vi "BCU参数读取-Auto.vi"(8 "CAN端口":u16(ring), 9 "设备索引号":u16(ring), 10 "CAN卡类型":u32(ring)=21, 11 "Myindex":dbl=1.0) -> (3 "成功":bool)   [LabVIEW 2013] (continued)
                      n2808 = property class="Tbl (严格)"(reference=w4454, "Active Cell"=w4453, "Cell BG Color"=u32 6618880) -> ()  [unwired: 1 in, 2 out]
                    }
                  }
                }
                n2809 = Select(t=0, s=w4406, f=1) -> (s? t:f=w4405:i32)
                n2810 = property on="从板个数" class="DigNum (严格)"("NumText.BGColor"=u32 13816530) -> ()  [unwired: 2 in, 2 out]
                n2811 = property on="项目信息" class="Tbl (严格)"("Disabled"=w4405) -> ()  [unwired: 2 in, 2 out]
                n2812 = global read "功能码全局.vi" "主板项目信息5"() -> (w4413:bool[])
                n2813 = global read "功能码全局.vi" "主板项目信息6"() -> (w4411:bool[])
                n2814 = Index Array(array=w4413, index=5 ("索引")) -> (element=w4410:bool)
                n2815 = Index Array(array=w4411, index=6 ("索引")) -> (element=w4409:bool)
                n2816 = Not(x=w4419) -> (.not. x?=w4418:bool)
              }
              frame "保险位置" {
                w4467 = 2
                w4469 = FALSE
                n2817 = property on="电池实际容量(A)" class="DigNum (严格)"("Disabled"=w4467) -> ()  [unwired: 2 in, 2 out]
                n2818 = property on="使用者" class="DigNum (严格)"("Disabled"=w4467) -> ()  [unwired: 2 in, 2 out]
                n2819 = property on="SOH(%)" class="DigNum (严格)"("Disabled"=w4467) -> ()  [unwired: 2 in, 2 out]
                n2820 = property on="电池额定容量(A)" class="DigNum (严格)"("Disabled"=w4467) -> ()  [unwired: 2 in, 2 out]
                n2821 = property on="SOC(%)" class="DigNum (严格)"("Disabled"=w4467) -> ()  [unwired: 2 in, 2 out]
                n2822 = local read "从板个数"() -> (w4465:dbl)
                n2823 = property on="系统时钟" class="Str"("Disabled"=w4467) -> ()  [unwired: 2 in, 2 out]
                n2824 = property on="配置文件版本" class="Str"("Disabled"=w4467) -> ()  [unwired: 2 in, 2 out]
                n2825 = property on="车架(牌)号" class="Str"("Disabled"=w4467) -> ()  [unwired: 2 in, 2 out]
                n2826 = property on="产品编号" class="Str"("Disabled"=w4467) -> ()  [unwired: 2 in, 2 out]
                n2827 = control-ref of="项目信息"() -> (w4466:refnum<vi>)
                n2828 = stacked-sequence {
                  tunnel: w4466 -> [w4478 w4481]
                  tunnel: w4465 -> [w4471 w4480]
                  frame #0 {
                    n2829 = Multiply(x=w4471, y=4.0) -> (x*y=w4473:dbl)
                    n2830 = Compound Arithmetic op=ADD(24.0 ("值"), w4473) -> (w4475:dbl)
                    n2831 = Bundle(w4475, 0) -> (w4477:cluster{dbl, i32})  [unwired: 1 out]
                    n2832 = property class="Tbl (严格)"(reference=w4478, "Index Values"=w4477) -> ()  [unwired: 1 in, 2 out]
                  }
                  frame #1 {
                    n2833 = for {
                      N: 20 -> [_]
                      tunnel: w4481 -> [w4491]
                      tunnel: w4480 -> [w4486]
                      i -> [w4485]
                      n2834 = Multiply(x=4.0, y=w4486) -> (x*y=w4483:dbl)
                      n2835 = Compound Arithmetic op=ADD(24.0 ("值"), w4483, w4485) -> (w4488:dbl)
                      n2836 = Bundle(w4488, 0) -> (w4490:cluster{dbl, i32})  [unwired: 1 out]
                      n2837 = property class="Tbl (严格)"(reference=w4491, "Active Cell"=w4490, "Cell BG Color"=u32 6618880) -> ()  [unwired: 1 in, 2 out]
                    }
                  }
                }
                n2838 = property on="从板个数" class="DigNum (严格)"("NumText.BGColor"=u32 13816530) -> ()  [unwired: 2 in, 2 out]
                n2839 = Select(t=0, s=w4458, f=1) -> (s? t:f=w4456:i32)
                n2840 = global read "功能码全局.vi" "主板项目信息4"() -> (w4463:bool[])
                n2841 = property on="项目信息" class="Tbl (严格)"("Disabled"=w4456) -> ()  [unwired: 2 in, 2 out]
                n2842 = Index Array(array=w4463, index #1=5 ("索引"), index #2=6 ("索引")) -> (element #1=w4461:bool, element #2=w4460:bool)
                n2843 = Not(x=w4469) -> (.not. x?=w4468:bool)
              }
              frame "SOC" {
                w4502 = 2
                w4504 = FALSE
                n2844 = property on="电池实际容量(A)" class="DigNum (严格)"("Disabled"=w4502) -> ()  [unwired: 2 in, 2 out]
                n2845 = property on="使用者" class="DigNum (严格)"("Disabled"=w4502) -> ()  [unwired: 2 in, 2 out]
                n2846 = property on="SOH(%)" class="DigNum (严格)"("Disabled"=w4502) -> ()  [unwired: 2 in, 2 out]
                n2847 = property on="电池额定容量(A)" class="DigNum (严格)"("Disabled"=w4502) -> ()  [unwired: 2 in, 2 out]
                n2848 = property on="从板个数" class="DigNum (严格)"("NumText.BGColor"=u32 13816530) -> ()  [unwired: 2 in, 2 out]
                n2849 = property on="系统时钟" class="Str"("Disabled"=w4502) -> ()  [unwired: 2 in, 2 out]
                n2850 = property on="配置文件版本" class="Str"("Disabled"=w4502) -> ()  [unwired: 2 in, 2 out]
                n2851 = property on="车架(牌)号" class="Str"("Disabled"=w4502) -> ()  [unwired: 2 in, 2 out]
                n2852 = property on="项目信息" class="Tbl (严格)"("Disabled"=w4502) -> ()  [unwired: 2 in, 2 out]
                n2853 = property on="产品编号" class="Str"("Disabled"=w4502) -> ()  [unwired: 2 in, 2 out]
                n2854 = Select(t=0, s=w4494, f=0) -> (s? t:f=w4493:i32)
                n2855 = property on="SOC(%)" class="DigNum (严格)"("Disabled"=w4493) -> ()  [unwired: 2 in, 2 out]
                n2856 = property on="项目信息2" class="Clust (严格)"("DisabledEnum"=w4493) -> ()  [unwired: 2 in, 2 out]
                n2857 = global read "功能码全局.vi" "主板项目信息7"() -> (w4500:bool[])
                n2858 = Index Array(array=w4500, index #1=2 ("索引"), index #2=5 ("索引")) -> (element #1=w4498:bool, element #2=w4497:bool)
                n2859 = Not(x=w4504) -> (.not. x?=w4503:bool)
              }
              frame "电池额定实际容量" {
                w4516 = 2
                w4518 = FALSE
                n2860 = property on="使用者" class="DigNum (严格)"("Disabled"=w4516) -> ()  [unwired: 2 in, 2 out]
                n2861 = property on="SOH(%)" class="DigNum (严格)"("Disabled"=w4516) -> ()  [unwired: 2 in, 2 out]
                n2862 = property on="SOC(%)" class="DigNum (严格)"("Disabled"=w4516) -> ()  [unwired: 2 in, 2 out]
                n2863 = property on="从板个数" class="DigNum (严格)"("NumText.BGColor"=u32 13816530) -> ()  [unwired: 2 in, 2 out]
                n2864 = property on="系统时钟" class="Str"("Disabled"=w4516) -> ()  [unwired: 2 in, 2 out]
                n2865 = property on="配置文件版本" class="Str"("Disabled"=w4516) -> ()  [unwired: 2 in, 2 out]
                n2866 = property on="车架(牌)号" class="Str"("Disabled"=w4516) -> ()  [unwired: 2 in, 2 out]
                n2867 = property on="项目信息" class="Tbl (严格)"("Disabled"=w4516) -> ()  [unwired: 2 in, 2 out]
                n2868 = property on="产品编号" class="Str"("Disabled"=w4516) -> ()  [unwired: 2 in, 2 out]
                n2869 = Select(t=0, s=w4508, f=1) -> (s? t:f=w4507:i32)
                n2870 = property on="电池实际容量(A)" class="DigNum (严格)"("Disabled"=w4507) -> ()  [unwired: 2 in, 2 out]
                n2871 = property on="电池额定容量(A)" class="DigNum (严格)"("Disabled"=w4507) -> ()  [unwired: 2 in, 2 out]
                n2872 = property on="项目信息2" class="Clust (严格)"("DisabledEnum"=w4507) -> ()  [unwired: 2 in, 2 out]
                n2873 = global read "功能码全局.vi" "主板项目信息7"() -> (w4514:bool[])
                n2874 = Index Array(array=w4514, index #1=3 ("索引"), index #2=6 ("索引")) -> (element #1=w4512:bool, element #2=w4511:bool)
                n2875 = Not(x=w4518) -> (.not. x?=w4517:bool)
              }
              frame "配置文件版本" {
                w4531 = 2
                w4533 = FALSE
                n2876 = property on="使用者" class="DigNum (严格)"("Disabled"=w4531) -> ()  [unwired: 2 in, 2 out]
                n2877 = property on="SOH(%)" class="DigNum (严格)"("Disabled"=w4531) -> ()  [unwired: 2 in, 2 out]
                n2878 = property on="SOC(%)" class="DigNum (严格)"("Disabled"=w4531) -> ()  [unwired: 2 in, 2 out]
                n2879 = property on="电池实际容量(A)" class="DigNum (严格)"("Disabled"=w4531) -> ()  [unwired: 2 in, 2 out]
                n2880 = property on="从板个数" class="DigNum (严格)"("NumText.BGColor"=u32 13816530) -> ()  [unwired: 2 in, 2 out]
                n2881 = property on="电池额定容量(A)" class="DigNum (严格)"("Disabled"=w4531) -> ()  [unwired: 2 in, 2 out]
                n2882 = property on="系统时钟" class="Str"("Disabled"=w4531) -> ()  [unwired: 2 in, 2 out]
                n2883 = property on="车架(牌)号" class="Str"("Disabled"=w4531) -> ()  [unwired: 2 in, 2 out]
                n2884 = property on="项目信息" class="Tbl (严格)"("Disabled"=w4531) -> ()  [unwired: 2 in, 2 out]
                n2885 = property on="产品编号" class="Str"("Disabled"=w4531) -> ()  [unwired: 2 in, 2 out]
                n2886 = Select(t=0, s=w4522, f=1) -> (s? t:f=w4521:i32)
                n2887 = property on="项目信息2" class="Clust (严格)"("DisabledEnum"=w4521) -> ()  [unwired: 2 in, 2 out]
                n2888 = property on="配置文件版本" class="Str"("Disabled"=w4521) -> ()  [unwired: 2 in, 2 out]
                n2889 = global read "功能码全局.vi" "主板项目信息5"() -> (w4529:bool[])
                n2890 = global read "功能码全局.vi" "主板项目信息6"() -> (w4528:bool[])
                n2891 = Index Array(array=w4529, index=6 ("索引")) -> (element=w4526:bool)
                n2892 = Index Array(array=w4528, index=7 ("索引")) -> (element=w4525:bool)
                n2893 = Not(x=w4533) -> (.not. x?=w4532:bool)
              }
              frame "参数修改记录" {
                w4546 = 2
                w4548 = FALSE
                n2894 = property on="SOH(%)" class="DigNum (严格)"("Disabled"=w4546) -> ()  [unwired: 2 in, 2 out]
                n2895 = property on="SOC(%)" class="DigNum (严格)"("Disabled"=w4546) -> ()  [unwired: 2 in, 2 out]
                n2896 = property on="电池实际容量(A)" class="DigNum (严格)"("Disabled"=w4546) -> ()  [unwired: 2 in, 2 out]
                n2897 = property on="电池额定容量(A)" class="DigNum (严格)"("Disabled"=w4546) -> ()  [unwired: 2 in, 2 out]
                n2898 = property on="从板个数" class="DigNum (严格)"("NumText.BGColor"=u32 13816530) -> ()  [unwired: 2 in, 2 out]
                n2899 = property on="系统时钟" class="Str"("Disabled"=w4546) -> ()  [unwired: 2 in, 2 out]
                n2900 = property on="车架(牌)号" class="Str"("Disabled"=w4546) -> ()  [unwired: 2 in, 2 out]
                n2901 = property on="配置文件版本" class="Str"("Disabled"=w4546) -> ()  [unwired: 2 in, 2 out]
                n2902 = property on="项目信息" class="Tbl (严格)"("Disabled"=w4546) -> ()  [unwired: 2 in, 2 out]
                n2903 = property on="产品编号" class="Str"("Disabled"=w4546) -> ()  [unwired: 2 in, 2 out]
                n2904 = Select(t=0, s=w4537, f=1) -> (s? t:f=w4536:i32)
                n2905 = property on="使用者" class="DigNum (严格)"("Disabled"=w4536) -> ()  [unwired: 2 in, 2 out]
                n2906 = property on="项目信息2" class="Clust (严格)"("DisabledEnum"=w4536) -> ()  [unwired: 2 in, 2 out]
                n2907 = global read "功能码全局.vi" "主板项目信息7"() -> (w4543:bool[])
                n2908 = global read "功能码全局.vi" "主板项目信息5"() -> (w4544:bool[])
                n2909 = Index Array(array=w4543, index=0 ("索引")) -> (element=w4541:bool)
                n2910 = Index Array(array=w4544, index=7 ("索引")) -> (element=w4540:bool)
                n2911 = Not(x=w4548) -> (.not. x?=w4547:bool)
              }
              frame "车牌号" {
                w4561 = 2
                w4563 = FALSE
                n2912 = property on="SOH(%)" class="DigNum (严格)"("Disabled"=w4561) -> ()  [unwired: 2 in, 2 out]
                n2913 = property on="使用者" class="DigNum (严格)"("Disabled"=w4561) -> ()  [unwired: 2 in, 2 out]
                n2914 = property on="SOC(%)" class="DigNum (严格)"("Disabled"=w4561) -> ()  [unwired: 2 in, 2 out]
                n2915 = property on="电池实际容量(A)" class="DigNum (严格)"("Disabled"=w4561) -> ()  [unwired: 2 in, 2 out]
                n2916 = property on="电池额定容量(A)" class="DigNum (严格)"("Disabled"=w4561) -> ()  [unwired: 2 in, 2 out]
                n2917 = property on="从板个数" class="DigNum (严格)"("NumText.BGColor"=u32 13816530) -> ()  [unwired: 2 in, 2 out]
                n2918 = property on="系统时钟" class="Str"("Disabled"=w4561) -> ()  [unwired: 2 in, 2 out]
                n2919 = property on="配置文件版本" class="Str"("Disabled"=w4561) -> ()  [unwired: 2 in, 2 out]
                n2920 = property on="项目信息" class="Tbl (严格)"("Disabled"=w4561) -> ()  [unwired: 2 in, 2 out]
                n2921 = property on="产品编号" class="Str"("Disabled"=w4561) -> ()  [unwired: 2 in, 2 out]
                n2922 = Select(t=0, s=w4552, f=1) -> (s? t:f=w4551:i32)
                n2923 = property on="车架(牌)号" class="Str"("Disabled"=w4551) -> ()  [unwired: 2 in, 2 out]
                n2924 = property on="项目信息2" class="Clust (严格)"("DisabledEnum"=w4551) -> ()  [unwired: 2 in, 2 out]
                n2925 = global read "功能码全局.vi" "主板项目信息7"() -> (w4558:bool[])
                n2926 = global read "功能码全局.vi" "主板项目信息6"() -> (w4559:bool[])
                n2927 = Index Array(array=w4558, index=1 ("索引")) -> (element=w4556:bool)
                n2928 = Index Array(array=w4559, index=0 ("索引")) -> (element=w4555:bool)
                n2929 = Not(x=w4563) -> (.not. x?=w4562:bool)
              }
              frame "SOH" {
                w4575 = 2
                w4577 = FALSE
                n2930 = property on="使用者" class="DigNum (严格)"("Disabled"=w4575) -> ()  [unwired: 2 in, 2 out]
                n2931 = property on="SOC(%)" class="DigNum (严格)"("Disabled"=w4575) -> ()  [unwired: 2 in, 2 out]
                n2932 = property on="电池实际容量(A)" class="DigNum (严格)"("Disabled"=w4575) -> ()  [unwired: 2 in, 2 out]
                n2933 = property on="电池额定容量(A)" class="DigNum (严格)"("Disabled"=w4575) -> ()  [unwired: 2 in, 2 out]
                n2934 = property on="从板个数" class="DigNum (严格)"("NumText.BGColor"=u32 13816530) -> ()  [unwired: 2 in, 2 out]
                n2935 = property on="系统时钟" class="Str"("Disabled"=w4575) -> ()  [unwired: 2 in, 2 out]
                n2936 = property on="配置文件版本" class="Str"("Disabled"=w4575) -> ()  [unwired: 2 in, 2 out]
                n2937 = property on="项目信息" class="Tbl (严格)"("Disabled"=w4575) -> ()  [unwired: 2 in, 2 out]
                n2938 = property on="产品编号" class="Str"("Disabled"=w4575) -> ()  [unwired: 2 in, 2 out]
                n2939 = property on="车架(牌)号" class="Str"("Disabled"=w4575) -> ()  [unwired: 2 in, 2 out]
                n2940 = Select(t=0, s=w4567, f=1) -> (s? t:f=w4566:i32)
                n2941 = property on="项目信息2" class="Clust (严格)"("DisabledEnum"=w4566) -> ()  [unwired: 2 in, 2 out]
                n2942 = property on="SOH(%)" class="DigNum (严格)"("Disabled"=w4566) -> ()  [unwired: 2 in, 2 out]
                n2943 = global read "功能码全局.vi" "主板项目信息7"() -> (w4574:bool[])
                n2944 = Index Array(array=w4574, index #1=4 ("索引"), index #2=7 ("索引")) -> (element #1=w4571:bool, element #2=w4570:bool)
                n2945 = Not(x=w4577) -> (.not. x?=w4576:bool)
              }
              frame "SOC过低(2)", "SOC过高(2)", "SOH过低(2)", "充电电流过高(2)", "单体电压过低(2)", "单体电压过高(2)", "单组电压不均衡(2)", "单组温度不均衡(2)", "二级故障阀值", "放电电流过高(2)", "极柱温度过高(2)", "内阻过大(2)", "温度过低(2)", "温度过高(2)", "整组电压不均衡(2)", "整组温度不均衡(2)", "总电压过低(2)", "总电压过高(2)" {
                w4589 = FALSE
                n2946 = property on="从板个数" class="DigNum (严格)"("NumText.BGColor"=u32 13816530) -> ()  [unwired: 2 in, 2 out]
                n2947 = Select(t=0, s=w4581, f=1) -> (s? t:f=w4580:i32)
                n2948 = property on="一级故障 2" class="Clust (严格)"("DisabledEnum"=w4580) -> ()  [unwired: 2 in, 2 out]
                n2949 = global read "功能码全局.vi" "主板故障阀值9"() -> (w4587:bool[])
                n2950 = Index Array(array=w4587, index #1=3 ("索引"), index #2=6 ("索引")) -> (element #1=w4585:bool, element #2=w4584:bool)
                n2951 = Not(x=w4589) -> (.not. x?=w4590:bool)
              }
              frame "SOC过低(3)", "SOC过高(3)", "SOH过低(3)", "充电电流过高(3)", "单体电压过低(3)", "单体电压过高(3)", "单组电压不均衡(3)", "单组温度不均衡(3)", "放电电流过高(3)", "极柱温度过高(3)", "内阻过大(3)", "三级故障阀值", "温度过低(3)", "温度过高(3)", "整组电压不均衡(3)", "整组温度不均衡(3)", "总电压过低(3)", "总电压过高(3)" {
                w4603 = FALSE
                n2952 = property on="从板个数" class="DigNum (严格)"("NumText.BGColor"=u32 13816530) -> ()  [unwired: 2 in, 2 out]
                n2953 = Select(t=0, s=w4594, f=1) -> (s? t:f=w4593:i32)
                n2954 = property on="一级故障 3" class="Clust (严格)"("DisabledEnum"=w4593) -> ()  [unwired: 2 in, 2 out]
                n2955 = global read "功能码全局.vi" "主板故障阀值9"() -> (w4600:bool[])
                n2956 = Index Array(array=w4600, index #1=4 ("索引"), index #2=7 ("索引")) -> (element #1=w4598:bool, element #2=w4597:bool)
                n2957 = Not(x=w4603) -> (.not. x?=w4602:bool)
              }
              frame "SOC过低", "SOC过高", "SOH过低", "充电电流过高", "单体电压过低", "单体电压过高", "单组电压不均衡", "单组温度不均衡", "放电电流过高", "极柱温度过高", "内阻过大", "温度过低", "温度过高", "一级故障阀值", "整组电压不均衡", "整组温度不均衡", "总电压过低", "总电压过高" {
                w4616 = FALSE
                n2958 = Select(t=0, s=w4607, f=1) -> (s? t:f=w4606:i32)
                n2959 = property on="从板个数" class="DigNum (严格)"("NumText.BGColor"=u32 13816530) -> ()  [unwired: 2 in, 2 out]
                n2960 = property on="一级故障" class="Clust (严格)"("DisabledEnum"=w4606) -> ()  [unwired: 2 in, 2 out]
                n2961 = global read "功能码全局.vi" "主板故障阀值9"() -> (w4613:bool[])
                n2962 = Index Array(array=w4613, index #1=2 ("索引"), index #2=5 ("索引")) -> (element #1=w4611:bool, element #2=w4610:bool)
                n2963 = Not(x=w4616) -> (.not. x?=w4615:bool)
              }
              frame "充电控制参数", "电流步长", "最大允许充电电流", "最大允许充电温度", "最大允许单体电压", "最大允许总电压", "最小允许充电电流", "最小允许充电温度", "最小允许单体电压" {
                w4619 = 2
                w4630 = FALSE
                n2964 = property on="从板个数" class="DigNum (严格)"("NumText.BGColor"=u32 13816530) -> ()  [unwired: 2 in, 2 out]
                n2965 = property on="风机开启温度" class="DigNum (严格)"("Disabled"=w4619) -> ()  [unwired: 2 in, 2 out]
                n2966 = property on="风机关闭温度" class="DigNum (严格)"("Disabled"=w4619) -> ()  [unwired: 2 in, 2 out]
                n2967 = property on="加热开启温度" class="DigNum (严格)"("Disabled"=w4619) -> ()  [unwired: 2 in, 2 out]
                n2968 = property on="加热关闭温度" class="DigNum (严格)"("Disabled"=w4619) -> ()  [unwired: 2 in, 2 out]
                n2969 = property on="风机开启温差" class="DigNum (严格)"("Disabled"=w4619) -> ()  [unwired: 2 in, 2 out]
                n2970 = property on="风机关闭温差" class="DigNum (严格)"("Disabled"=w4619) -> ()  [unwired: 2 in, 2 out]
                n2971 = property on="加热控制参数" class="Clust (严格)"("DisabledEnum"=w4619) -> ()  [unwired: 2 in, 2 out]
                n2972 = Select(t=0, s=w4621, f=1) -> (s? t:f=w4620:i32)
                n2973 = property on="最大允许总电压" class="DigNum (严格)"("Disabled"=w4620) -> ()  [unwired: 2 in, 2 out]
                n2974 = property on="最大允许充电温度" class="DigNum (严格)"("Disabled"=w4620) -> ()  [unwired: 2 in, 2 out]
                n2975 = property on="最小允许充电温度" class="DigNum (严格)"("Disabled"=w4620) -> ()  [unwired: 2 in, 2 out]
                n2976 = property on="电流步长" class="DigNum (严格)"("Disabled"=w4620) -> ()  [unwired: 2 in, 2 out]
                n2977 = property on="最大允许单体电压" class="DigNum (严格)"("Disabled"=w4620) -> ()  [unwired: 2 in, 2 out]
                n2978 = property on="最小允许单体电压" class="DigNum (严格)"("Disabled"=w4620) -> ()  [unwired: 2 in, 2 out]
                n2979 = property on="最大允许充电电流" class="DigNum (严格)"("Disabled"=w4620) -> ()  [unwired: 2 in, 2 out]
                n2980 = property on="最小允许充电电流" class="DigNum (严格)"("Disabled"=w4620) -> ()  [unwired: 2 in, 2 out]
                n2981 = global read "功能码全局.vi" "主板控制类信息10"() -> (w4627:bool[])
                n2982 = Index Array(array=w4627, index #1=5 ("索引"), index #2=7 ("索引")) -> (element #1=w4625:bool, element #2=w4624:bool)
                n2983 = Not(x=w4630) -> (.not. x?=w4629:bool)
              }
              frame "风机关闭温差", "风机关闭温度", "风机开启温差", "风机开启温度", "加热关闭温差", "加热关闭温度", "加热开启温度", "加热控制参数" {
                w4642 = 2
                w4644 = FALSE
                n2984 = Select(t=0, s=w4634, f=1) -> (s? t:f=w4633:i32)
                n2985 = property on="从板个数" class="DigNum (严格)"("NumText.BGColor"=u32 13816530) -> ()  [unwired: 2 in, 2 out]
                n2986 = property on="加热控制参数" class="Clust (严格)"("DisabledEnum"=w4633) -> ()  [unwired: 2 in, 2 out]
                n2987 = property on="风机开启温度" class="DigNum (严格)"("Disabled"=w4633) -> ()  [unwired: 2 in, 2 out]
                n2988 = property on="风机关闭温度" class="DigNum (严格)"("Disabled"=w4633) -> ()  [unwired: 2 in, 2 out]
                n2989 = property on="加热开启温度" class="DigNum (严格)"("Disabled"=w4633) -> ()  [unwired: 2 in, 2 out]
                n2990 = property on="加热关闭温度" class="DigNum (严格)"("Disabled"=w4633) -> ()  [unwired: 2 in, 2 out]
                n2991 = property on="风机开启温差" class="DigNum (严格)"("Disabled"=w4633) -> ()  [unwired: 2 in, 2 out]
                n2992 = property on="风机关闭温差" class="DigNum (严格)"("Disabled"=w4633) -> ()  [unwired: 2 in, 2 out]
                n2993 = property on="最大允许总电压" class="DigNum (严格)"("Disabled"=w4642) -> ()  [unwired: 2 in, 2 out]
                n2994 = property on="最大允许充电温度" class="DigNum (严格)"("Disabled"=w4642) -> ()  [unwired: 2 in, 2 out]
                n2995 = property on="最小允许充电温度" class="DigNum (严格)"("Disabled"=w4642) -> ()  [unwired: 2 in, 2 out]
                n2996 = property on="电流步长" class="DigNum (严格)"("Disabled"=w4642) -> ()  [unwired: 2 in, 2 out]
                n2997 = property on="最大允许单体电压" class="DigNum (严格)"("Disabled"=w4642) -> ()  [unwired: 2 in, 2 out]
                n2998 = property on="最小允许单体电压" class="DigNum (严格)"("Disabled"=w4642) -> ()  [unwired: 2 in, 2 out]
                n2999 = property on="最大允许充电电流" class="DigNum (严格)"("Disabled"=w4642) -> ()  [unwired: 2 in, 2 out]
                n3000 = property on="最小允许充电电流" class="DigNum (严格)"("Disabled"=w4642) -> ()  [unwired: 2 in, 2 out]
                n3001 = global read "功能码全局.vi" "主板控制类信息10"() -> (w4640:bool[])
                n3002 = Index Array(array=w4640, index #1=4 ("索引"), index #2=6 ("索引")) -> (element #1=w4638:bool, element #2=w4637:bool)
                n3003 = Not(x=w4644) -> (.not. x?=w4643:bool)
              }
              frame "电池信息" {
                w4657 = FALSE
                n3004 = Select(t=0, s=w4648, f=1) -> (s? t:f=w4647:i32)
                n3005 = property on="电池串联" class="DigNum (严格)"("Disabled"=w4647) -> ()  [unwired: 2 in, 2 out]
                n3006 = property on="电池并联" class="DigNum (严格)"("Disabled"=w4647) -> ()  [unwired: 2 in, 2 out]
                n3007 = property on="电池包额定容量" class="DigNum (严格)"("Disabled"=w4647) -> ()  [unwired: 2 in, 2 out]
                n3008 = property on="电池包额定能量(kWh)" class="DigNum (严格)"("Disabled"=w4647) -> ()  [unwired: 2 in, 2 out]
                n3009 = property on="电池包额定总电压" class="DigNum (严格)"("Disabled"=w4647) -> ()  [unwired: 2 in, 2 out]
                n3010 = property on="实际容量" class="DigNum (严格)"("Disabled"=w4647) -> ()  [unwired: 2 in, 2 out]
                n3011 = property on="电池包组号" class="Str"("Disabled"=w4647) -> ()  [unwired: 2 in, 2 out]
                n3012 = property on="电池生产日期" class="Str"("Disabled"=w4647) -> ()  [unwired: 2 in, 2 out]
                n3013 = property on="电池厂家" class="Str"("Disabled"=w4647) -> ()  [unwired: 2 in, 2 out]
                n3014 = property on="电池类型" class="Str"("Disabled"=w4647) -> ()  [unwired: 2 in, 2 out]
                n3015 = property on="累计充电总安时" class="DigNum (严格)"("Disabled"=w4647) -> ()  [unwired: 2 in, 2 out]
                n3016 = property on="累计放电总安时" class="DigNum (严格)"("Disabled"=w4647) -> ()  [unwired: 2 in, 2 out]
                n3017 = property on="电池放空次数" class="DigNum (严格)"("Disabled"=w4647) -> ()  [unwired: 2 in, 2 out]
                n3018 = property on="电池充满次数" class="DigNum (严格)"("Disabled"=w4647) -> ()  [unwired: 2 in, 2 out]
                n3019 = property on="电池充电次数" class="DigNum (严格)"("Disabled"=w4647) -> ()  [unwired: 2 in, 2 out]
                n3020 = property on="电池信息" class="Clust (严格)"("DisabledEnum"=w4647) -> ()  [unwired: 2 in, 2 out]
                n3021 = global read "功能码全局.vi" "主板版本号11"() -> (w4654:bool[])
                n3022 = property on="从板个数" class="DigNum (严格)"("NumText.BGColor"=u32 13816530) -> ()  [unwired: 2 in, 2 out]
                n3023 = Index Array(array=w4654, index #1=0 ("索引"), index #2=1 ("索引")) -> (element #1=w4652:bool, element #2=w4651:bool)
                n3024 = Not(x=w4657) -> (.not. x?=w4656:bool)
              }
              frame "电池信息1" {
                w4669 = 2
                w4671 = FALSE
                n3025 = Select(t=0, s=w4661, f=1) -> (s? t:f=w4660:i32)
                n3026 = property on="电池信息" class="Clust (严格)"("DisabledEnum"=w4660) -> ()  [unwired: 2 in, 2 out]
                n3027 = property on="电池生产日期" class="Str"("Disabled"=w4660) -> ()  [unwired: 2 in, 2 out]
                n3028 = property on="电池厂家" class="Str"("Disabled"=w4660) -> ()  [unwired: 2 in, 2 out]
                n3029 = property on="电池类型" class="Str"("Disabled"=w4660) -> ()  [unwired: 2 in, 2 out]
                n3030 = property on="电池串联" class="DigNum (严格)"("Disabled"=w4660) -> ()  [unwired: 2 in, 2 out]
                n3031 = property on="电池并联" class="DigNum (严格)"("Disabled"=w4660) -> ()  [unwired: 2 in, 2 out]
                n3032 = property on="电池包额定容量" class="DigNum (严格)"("Disabled"=w4660) -> ()  [unwired: 2 in, 2 out]
                n3033 = property on="电池包额定能量(kWh)" class="DigNum (严格)"("Disabled"=w4660) -> ()  [unwired: 2 in, 2 out]
                n3034 = property on="电池包额定总电压" class="DigNum (严格)"("Disabled"=w4660) -> ()  [unwired: 2 in, 2 out]
                n3035 = property on="实际容量" class="DigNum (严格)"("Disabled"=w4660) -> ()  [unwired: 2 in, 2 out]
                n3036 = property on="累计充电总安时" class="DigNum (严格)"("Disabled"=w4669) -> ()  [unwired: 2 in, 2 out]
                n3037 = property on="累计放电总安时" class="DigNum (严格)"("Disabled"=w4669) -> ()  [unwired: 2 in, 2 out]
                n3038 = property on="电池放空次数" class="DigNum (严格)"("Disabled"=w4669) -> ()  [unwired: 2 in, 2 out]
                n3039 = property on="电池充满次数" class="DigNum (严格)"("Disabled"=w4669) -> ()  [unwired: 2 in, 2 out]
                n3040 = property on="电池充电次数" class="DigNum (严格)"("Disabled"=w4669) -> ()  [unwired: 2 in, 2 out]
                n3041 = property on="从板个数" class="DigNum (严格)"("NumText.BGColor"=u32 13816530) -> ()  [unwired: 2 in, 2 out]
                n3042 = property on="电池包组号" class="Str"("Disabled"=w4669) -> ()  [unwired: 2 in, 2 out]
                n3043 = global read "功能码全局.vi" "主板版本号11"() -> (w4667:bool[])
                n3044 = Index Array(array=w4667, index #1=0 ("索引"), index #2=1 ("索引")) -> (element #1=w4665:bool, element #2=w4664:bool)
                n3045 = Not(x=w4671) -> (.not. x?=w4670:bool)
              }
              frame "电池包组号" {
                w4683 = 2
                w4685 = FALSE
                n3046 = property on="电池生产日期" class="Str"("Disabled"=w4683) -> ()  [unwired: 2 in, 2 out]
                n3047 = property on="电池厂家" class="Str"("Disabled"=w4683) -> ()  [unwired: 2 in, 2 out]
                n3048 = property on="电池类型" class="Str"("Disabled"=w4683) -> ()  [unwired: 2 in, 2 out]
                n3049 = property on="电池串联" class="DigNum (严格)"("Disabled"=w4683) -> ()  [unwired: 2 in, 2 out]
                n3050 = property on="电池并联" class="DigNum (严格)"("Disabled"=w4683) -> ()  [unwired: 2 in, 2 out]
                n3051 = property on="电池包额定容量" class="DigNum (严格)"("Disabled"=w4683) -> ()  [unwired: 2 in, 2 out]
                n3052 = property on="电池包额定能量(kWh)" class="DigNum (严格)"("Disabled"=w4683) -> ()  [unwired: 2 in, 2 out]
                n3053 = property on="电池包额定总电压" class="DigNum (严格)"("Disabled"=w4683) -> ()  [unwired: 2 in, 2 out]
                n3054 = property on="实际容量" class="DigNum (严格)"("Disabled"=w4683) -> ()  [unwired: 2 in, 2 out]
                n3055 = property on="从板个数" class="DigNum (严格)"("NumText.BGColor"=u32 13816530) -> ()  [unwired: 2 in, 2 out]
                n3056 = property on="累计充电总安时" class="DigNum (严格)"("Disabled"=w4683) -> ()  [unwired: 2 in, 2 out]
                n3057 = property on="累计放电总安时" class="DigNum (严格)"("Disabled"=w4683) -> ()  [unwired: 2 in, 2 out]
                n3058 = property on="电池放空次数" class="DigNum (严格)"("Disabled"=w4683) -> ()  [unwired: 2 in, 2 out]
                n3059 = property on="电池充满次数" class="DigNum (严格)"("Disabled"=w4683) -> ()  [unwired: 2 in, 2 out]
                n3060 = property on="电池充电次数" class="DigNum (严格)"("Disabled"=w4683) -> ()  [unwired: 2 in, 2 out]
                n3061 = Select(t=0, s=w4675, f=1) -> (s? t:f=w4674:i32)
                n3062 = property on="电池包组号" class="Str"("Disabled"=w4674) -> ()  [unwired: 2 in, 2 out]
                n3063 = property on="电池信息" class="Clust (严格)"("DisabledEnum"=w4674) -> ()  [unwired: 2 in, 2 out]
                n3064 = global read "功能码全局.vi" "主板版本号11"() -> (w4681:bool[])
                n3065 = Index Array(array=w4681, index #1=0 ("索引"), index #2=1 ("索引")) -> (element #1=w4679:bool, element #2=w4678:bool)
                n3066 = Not(x=w4685) -> (.not. x?=w4684:bool)
              }
              frame "充放电安时" {
                w4697 = 2
                w4699 = FALSE
                n3067 = property on="电池生产日期" class="Str"("Disabled"=w4697) -> ()  [unwired: 2 in, 2 out]
                n3068 = property on="电池厂家" class="Str"("Disabled"=w4697) -> ()  [unwired: 2 in, 2 out]
                n3069 = property on="电池类型" class="Str"("Disabled"=w4697) -> ()  [unwired: 2 in, 2 out]
                n3070 = property on="电池串联" class="DigNum (严格)"("Disabled"=w4697) -> ()  [unwired: 2 in, 2 out]
                n3071 = property on="电池并联" class="DigNum (严格)"("Disabled"=w4697) -> ()  [unwired: 2 in, 2 out]
                n3072 = property on="电池包额定容量" class="DigNum (严格)"("Disabled"=w4697) -> ()  [unwired: 2 in, 2 out]
                n3073 = property on="电池包额定能量(kWh)" class="DigNum (严格)"("Disabled"=w4697) -> ()  [unwired: 2 in, 2 out]
                n3074 = property on="电池包额定总电压" class="DigNum (严格)"("Disabled"=w4697) -> ()  [unwired: 2 in, 2 out]
                n3075 = property on="实际容量" class="DigNum (严格)"("Disabled"=w4697) -> ()  [unwired: 2 in, 2 out]
                n3076 = property on="从板个数" class="DigNum (严格)"("NumText.BGColor"=u32 13816530) -> ()  [unwired: 2 in, 2 out]
                n3077 = Select(t=0, s=w4689, f=1) -> (s? t:f=w4688:i32)
                n3078 = property on="电池放空次数" class="DigNum (严格)"("Disabled"=w4697) -> ()  [unwired: 2 in, 2 out]
                n3079 = property on="电池充满次数" class="DigNum (严格)"("Disabled"=w4697) -> ()  [unwired: 2 in, 2 out]
                n3080 = property on="电池充电次数" class="DigNum (严格)"("Disabled"=w4697) -> ()  [unwired: 2 in, 2 out]
                n3081 = property on="电池包组号" class="Str"("Disabled"=w4697) -> ()  [unwired: 2 in, 2 out]
                n3082 = property on="累计充电总安时" class="DigNum (严格)"("Disabled"=w4688) -> ()  [unwired: 2 in, 2 out]
                n3083 = property on="累计放电总安时" class="DigNum (严格)"("Disabled"=w4688) -> ()  [unwired: 2 in, 2 out]
                n3084 = property on="电池信息" class="Clust (严格)"("DisabledEnum"=w4688) -> ()  [unwired: 2 in, 2 out]
                n3085 = global read "功能码全局.vi" "主板版本号11"() -> (w4695:bool[])
                n3086 = Index Array(array=w4695, index #1=0 ("索引"), index #2=1 ("索引")) -> (element #1=w4693:bool, element #2=w4692:bool)
                n3087 = Not(x=w4699) -> (.not. x?=w4698:bool)
              }
              frame "电池充放电次数" {
                w4711 = 2
                w4713 = FALSE
                n3088 = property on="从板个数" class="DigNum (严格)"("NumText.BGColor"=u32 13816530) -> ()  [unwired: 2 in, 2 out]
                n3089 = property on="电池生产日期" class="Str"("Disabled"=w4711) -> ()  [unwired: 2 in, 2 out]
                n3090 = property on="电池厂家" class="Str"("Disabled"=w4711) -> ()  [unwired: 2 in, 2 out]
                n3091 = property on="电池类型" class="Str"("Disabled"=w4711) -> ()  [unwired: 2 in, 2 out]
                n3092 = property on="电池串联" class="DigNum (严格)"("Disabled"=w4711) -> ()  [unwired: 2 in, 2 out]
                n3093 = property on="电池并联" class="DigNum (严格)"("Disabled"=w4711) -> ()  [unwired: 2 in, 2 out]
                n3094 = property on="电池包额定容量" class="DigNum (严格)"("Disabled"=w4711) -> ()  [unwired: 2 in, 2 out]
                n3095 = property on="电池包额定能量(kWh)" class="DigNum (严格)"("Disabled"=w4711) -> ()  [unwired: 2 in, 2 out]
                n3096 = property on="电池包额定总电压" class="DigNum (严格)"("Disabled"=w4711) -> ()  [unwired: 2 in, 2 out]
                n3097 = property on="实际容量" class="DigNum (严格)"("Disabled"=w4711) -> ()  [unwired: 2 in, 2 out]
                n3098 = Select(t=0, s=w4703, f=1) -> (s? t:f=w4702:i32)
                n3099 = property on="电池放空次数" class="DigNum (严格)"("Disabled"=w4702) -> ()  [unwired: 2 in, 2 out]
                n3100 = property on="电池充满次数" class="DigNum (严格)"("Disabled"=w4702) -> ()  [unwired: 2 in, 2 out]
                n3101 = property on="电池充电次数" class="DigNum (严格)"("Disabled"=w4702) -> ()  [unwired: 2 in, 2 out]
                n3102 = property on="累计充电总安时" class="DigNum (严格)"("Disabled"=w4711) -> ()  [unwired: 2 in, 2 out]
                n3103 = property on="累计放电总安时" class="DigNum (严格)"("Disabled"=w4711) -> ()  [unwired: 2 in, 2 out]
                n3104 = property on="电池信息" class="Clust (严格)"("DisabledEnum"=w4702) -> ()  [unwired: 2 in, 2 out]
                n3105 = property on="电池包组号" class="Str"("Disabled"=w4711) -> ()  [unwired: 2 in, 2 out]
                n3106 = global read "功能码全局.vi" "主板版本号11"() -> (w4709:bool[])
                n3107 = Index Array(array=w4709, index #1=0 ("索引"), index #2=1 ("索引")) -> (element #1=w4707:bool, element #2=w4706:bool)
                n3108 = Not(x=w4713) -> (.not. x?=w4712:bool)
              }
              frame "假", Default {
                w4718 = FALSE
                n3109 = Not(x=w4718) -> (.not. x?=w4717:bool)
              }
            }
            n3110 = property on="单个读取" class="Bool (严格)"("Visible"=w4186) -> ()  [unwired: 2 in, 2 out]
            n3111 = property on="单个写入" class="Bool (严格)"("Visible"=w4185) -> ()  [unwired: 2 in, 2 out]
            n3112 = local write "1"(w4193) -> ()
            n3113 = local write "1 2"(w4192) -> ()
            n3114 = local write "1 3"(w4191) -> ()
            n3115 = local write "1 4"(w4190) -> ()
            n3116 = local write "1 5"(w4189) -> ()
            n3117 = local write "1 11"(w4188) -> ()
            n3118 = local write "主板2"(w4194) -> ()
          }
          event "从板选项": Mouse Down {
            n3119 = event-data() -> ("CtlRef"=w4733:refnum<vi>)  [unwired: 8 out]
            n3120 = property class="Tree (严格)"(reference=w4733) -> ("Value"=w4732:string)  [unwired: 1 in, 2 out]
            n3121 = global read "功能码全局.vi" "主板监控2"() -> (w4723:bool[])
            n3122 = Index Array(array=w4723, index=6 ("索引")) -> (element=w4721:bool)
            n3123 = case shown="\"二维码\"" w4732 {
              tunnel: [T19."从板信息" ("等级 2") T19."从板信息" ("等级 2") T19."从板信息" ("等级 2") T19."从板信息" ("等级 2") T19."从板信息" ("等级 2") T19."从板信息" ("等级 2") T19."从板信息" ("等级 2") T19."从板信息" ("等级 2") T19."一级故障阀值" ("等级 2") T19."二级故障阀值" ("等级 2") T19."三级故障阀值" ("等级 2") T19."快换参数" ("等级 2") T19."快换参数" ("等级 2") T19."快换参数" ("等级 2") T19."快换参数" ("等级 2") T19."快换参数" ("等级 2") T19."快换参数" ("等级 2") T19."快换参数" ("等级 2") T19."快换参数" ("等级 2") T14."均衡参数" ("等级 2") T14."均衡参数" ("等级 2") T14."均衡参数" ("等级 2") T19."从板信息" ("等级 2")] -> w4731
              tunnel: [w4744 w4754 w4764 w4778 w4793 w4828 w4865 w4902 w4926 w4939 w4952 w4965 w4991 w5005 w5021 w5038 w5055 w5073 w5092 w5109 w5122 w5136 w5151] -> w4730
              tunnel: [w4736 w4746 w4756 w4766 w4780 w4815 w4852 w4889 w4937 w4939 w4952 w4965 w4991 w5005 w5021 w5038 w5055 w5073 w5092 w5109 w5122 w5136 w5150] -> w4729
              tunnel: [w4736 w4746 w4756 w4766 w4780 w4815 w4852 w4889 w4926 w4950 w4952 w4965 w4991 w5005 w5021 w5038 w5055 w5073 w5092 w5109 w5122 w5136 w5150] -> w4728
              tunnel: [w4736 w4746 w4756 w4766 w4780 w4815 w4852 w4889 w4926 w4939 w4963 w4965 w4991 w5005 w5021 w5038 w5055 w5073 w5092 w5109 w5122 w5136 w5150] -> w4727
              tunnel: [w4736 w4746 w4756 w4766 w4780 w4815 w4852 w4889 w4926 w4939 w4952 w4989 w5003 w5019 w5036 w5053 w5071 w5090 w5107 w5109 w5122 w5136 w5150] -> w4726
              tunnel: [w4741 w4751 w4757 w4773 w4787 w4822 w4859 w4896 w4933 w4946 w4959 w4974 w4996 w5011 w5025 w5043 w5058 w5078 w5096 w5112 w5126 w5141 w5150] -> w4725
              tunnel: [w4738 w4748 w4757 w4772 w4786 w4821 w4858 w4895 w4932 w4945 w4958 w4966 w4995 w5010 w5024 w5044 w5059 w5077 w5095 w5111 w5125 w5140 w5150] -> w4724
              tunnel: w4721 -> [_ _ w4761 w4769 w4783 w4818 w4855 w4892 w4928 w4942 w4955 w4986 w4999 w5014 w5029 w5047 w5063 w5081 w5100 w5115 w5129 w5143 _]
              tunnel: [w4736 w4746 w4756 w4766 w4780 w4815 w4852 w4889 w4926 w4939 w4952 w4965 w4991 w5005 w5021 w5038 w5055 w5073 w5092 w5110 w5123 w5137 w5150] -> w4720
              frame "从板号" {
                w4743 = 2
                w4736 = FALSE ("1 6")
                n3124 = property on="项目信息 2" class="Tbl (严格)"("Disabled"=w4743) -> ()  [unwired: 2 in, 2 out]
                n3125 = property on="加热控制参数" class="Clust (严格)"("Disabled"=w4743) -> ()  [unwired: 2 in, 2 out]
                n3126 = property on="从板号" class="DigNum (严格)"("NumText.BGColor"=u32 6618880) -> ()  [unwired: 2 in, 2 out]
                n3127 = global read "功能码全局.vi" "16"() -> (w4740:bool[])
                n3128 = Index Array(array=w4740, index #1=4 ("索引"), index #2=6 ("索引")) -> (element #1=w4741:bool, element #2=w4738:bool)
                n3129 = Not(x=w4736) -> (.not. x?=w4744:bool)
              }
              frame "二维码" {
                w4753 = 2
                w4746 = FALSE ("1 6")
                n3130 = property on="项目信息 2" class="Tbl (严格)"("Disabled"=w4753) -> ()  [unwired: 2 in, 2 out]
                n3131 = property on="加热控制参数" class="Clust (严格)"("Disabled"=w4753) -> ()  [unwired: 2 in, 2 out]
                n3132 = property on="从板号" class="DigNum (严格)"("NumText.BGColor"=u32 6618880) -> ()  [unwired: 2 in, 2 out]
                n3133 = global read "功能码全局.vi" "16"() -> (w4750:bool[])
                n3134 = Index Array(array=w4750, index #1=4 ("索引"), index #2=6 ("索引")) -> (element #1=w4751:bool, element #2=w4748:bool)
                n3135 = Not(x=w4746) -> (.not. x?=w4754:bool)
              }
              frame "从板信息" {
                w4756 = FALSE ("1 6")
                n3136 = Select(t=0, s=w4761, f=1) -> (s? t:f=w4760:i32)
                n3137 = property on="从板号" class="DigNum (严格)"("NumText.BGColor"=u32 16777215) -> ()  [unwired: 2 in, 2 out]
                n3138 = property on="项目信息 2" class="Tbl (严格)"("Disabled"=w4760) -> ()  [unwired: 2 in, 2 out]
                n3139 = property on="加热控制参数" class="Clust (严格)"("Disabled"=w4760) -> ()  [unwired: 2 in, 2 out]
                n3140 = Not(x=w4756) -> (.not. x?=w4764:bool)
                n3141 = local read "从板项目信息"() -> (w4758:bool)
                n3142 = Not(x=w4758) -> (.not. x?=w4757:bool)
              }
              frame "风机关闭温差", "风机关闭温度", "风机开启温差", "风机开启温度", "加热关闭温差", "加热关闭温度", "加热开启温度", "加热控制参数" {
                w4766 = FALSE ("1 6")
                n3143 = property on="从板号" class="DigNum (严格)"("NumText.BGColor"=u32 16777215) -> ()  [unwired: 2 in, 2 out]
                n3144 = Select(t=0, s=w4769, f=1) -> (s? t:f=w4768:i32)
                n3145 = property on="项目信息 2" class="Tbl (严格)"("Disabled"=2) -> ()  [unwired: 2 in, 2 out]
                n3146 = property on="加热控制参数" class="Clust (严格)"("Disabled"=w4768) -> ()  [unwired: 2 in, 2 out]
                n3147 = global read "功能码全局.vi" "16"() -> (w4775:bool[])
                n3148 = Index Array(array=w4775, index #1=5 ("索引"), index #2=7 ("索引")) -> (element #1=w4773:bool, element #2=w4772:bool)
                n3149 = Not(x=w4766) -> (.not. x?=w4778:bool)
              }
              frame "电压个数" {
                w4780 = FALSE ("1 6")
                n3150 = property on="从板号" class="DigNum (严格)"("NumText.BGColor"=u32 16777215) -> ()  [unwired: 2 in, 2 out]
                n3151 = control-ref of="项目信息 2"() -> (w4791:refnum<vi>)
                n3152 = stacked-sequence {
                  tunnel: w4791 -> [w4798 w4800 w4809]
                  frame #0 {
                    n3153 = Bundle(0, 0) -> (w4797:cluster{i32, i32})  [unwired: 1 out]
                    n3154 = property class="Tbl (严格)"(reference=w4798, "Index Values"=w4797) -> ()  [unwired: 1 in, 2 out]
                  }
                  frame #1 {
                    n3155 = for {
                      N: 40 -> [_]
                      tunnel: w4800 -> [w4807]
                      i -> [w4802]
                      n3156 = Compound Arithmetic op=ADD(0 ("值"), w4802) -> (w4804:i32)
                      n3157 = Bundle(w4804, 0) -> (w4806:cluster{i32, i32})  [unwired: 1 out]
                      n3158 = property class="Tbl (严格)"(reference=w4807, "Active Cell"=w4806, "Cell BG Color"=u32 16448250) -> ()  [unwired: 1 in, 2 out]
                    }
                  }
                  frame #2 {
                    n3159 = for {
                      N: 1 -> [_]
                      tunnel: w4809 -> [w4814]
                      i -> [w4810]
                      n3160 = Bundle(w4810, 0) -> (w4813:cluster{i32, i32})  [unwired: 1 out]
                      n3161 = property class="Tbl (严格)"(reference=w4814, "Active Cell"=w4813, "Cell BG Color"=u32 6618880) -> ()  [unwired: 1 in, 2 out]
                    }
                  }
                }
                n3162 = Select(t=0, s=w4783, f=1) -> (s? t:f=w4782:i32)
                n3163 = property on="项目信息 2" class="Tbl (严格)"("Disabled"=w4782) -> ()  [unwired: 2 in, 2 out]
                n3164 = property on="加热控制参数" class="Clust (严格)"("Disabled"=2) -> ()  [unwired: 2 in, 2 out]
                n3165 = global read "功能码全局.vi" "15"() -> (w4789:bool[])
                n3166 = Index Array(array=w4789, index #1=0 ("索引"), index #2=4 ("索引")) -> (element #1=w4787:bool, element #2=w4786:bool)
                n3167 = Not(x=w4780) -> (.not. x?=w4793:bool)
              }
              frame "通道电压节数" {
                w4815 = FALSE ("1 6")
                n3168 = property on="从板号" class="DigNum (严格)"("NumText.BGColor"=u32 16777215) -> ()  [unwired: 2 in, 2 out]
                n3169 = control-ref of="项目信息 2"() -> (w4826:refnum<vi>)
                n3170 = stacked-sequence {
                  tunnel: w4826 -> [w4833 w4835 w4844]
                  frame #0 {
                    n3171 = Bundle(22, 0) -> (w4832:cluster{i32, i32})  [unwired: 1 out]
                    n3172 = property class="Tbl (严格)"(reference=w4833, "Index Values"=w4832) -> ()  [unwired: 1 in, 2 out]
                  }
                  frame #1 {
                    n3173 = for {
                      N: 40 -> [_]
                      tunnel: w4835 -> [w4842]
                      i -> [w4837]
                      n3174 = Compound Arithmetic op=ADD(0 ("值"), w4837) -> (w4839:i32)
                      n3175 = Bundle(w4839, 0) -> (w4841:cluster{i32, i32})  [unwired: 1 out]
                      n3176 = property class="Tbl (严格)"(reference=w4842, "Active Cell"=w4841, "Cell BG Color"=u32 16448250) -> ()  [unwired: 1 in, 2 out]
                    }
                  }
                  frame #2 {
                    n3177 = for {
                      N: 5 -> [_]
                      tunnel: w4844 -> [w4851]
                      i -> [w4847]
                      n3178 = Add(x=22, y=w4847) -> (x+y=w4846:i32)
                      n3179 = Bundle(w4846, 0) -> (w4850:cluster{i32, i32})  [unwired: 1 out]
                      n3180 = property class="Tbl (严格)"(reference=w4851, "Active Cell"=w4850, "Cell BG Color"=u32 6618880) -> ()  [unwired: 1 in, 2 out]
                    }
                  }
                }
                n3181 = Select(t=0, s=w4818, f=1) -> (s? t:f=w4817:i32)
                n3182 = property on="项目信息 2" class="Tbl (严格)"("Disabled"=w4817) -> ()  [unwired: 2 in, 2 out]
                n3183 = property on="加热控制参数" class="Clust (严格)"("Disabled"=2) -> ()  [unwired: 2 in, 2 out]
                n3184 = global read "功能码全局.vi" "15"() -> (w4824:bool[])
                n3185 = Index Array(array=w4824, index #1=1 ("索引"), index #2=5 ("索引")) -> (element #1=w4822:bool, element #2=w4821:bool)
                n3186 = Not(x=w4815) -> (.not. x?=w4828:bool)
              }
              frame "保险位置" {
                w4852 = FALSE ("1 6")
                n3187 = control-ref of="项目信息 2"() -> (w4863:refnum<vi>)
                n3188 = stacked-sequence {
                  tunnel: w4863 -> [w4870 w4872 w4881]
                  frame #0 {
                    n3189 = Bundle(0, 0) -> (w4869:cluster{i32, i32})  [unwired: 1 out]
                    n3190 = property class="Tbl (严格)"(reference=w4870, "Index Values"=w4869) -> ()  [unwired: 1 in, 2 out]
                  }
                  frame #1 {
                    n3191 = for {
                      N: 40 -> [_]
                      tunnel: w4872 -> [w4879]
                      i -> [w4875]
                      n3192 = Add(x=2, y=w4875) -> (x+y=w4874:i32)
                      n3193 = Bundle(w4874, 0) -> (w4878:cluster{i32, i32})  [unwired: 1 out]
                      n3194 = property class="Tbl (严格)"(reference=w4879, "Active Cell"=w4878, "Cell BG Color"=u32 16448250) -> ()  [unwired: 1 in, 2 out]
                    }
                  }
                  frame #2 {
                    n3195 = for {
                      N: 20 -> [_]
                      tunnel: w4881 -> [w4888]
                      i -> [w4884]
                      n3196 = Add(x=2, y=w4884) -> (x+y=w4883:i32)
                      n3197 = Bundle(w4883, 0) -> (w4887:cluster{i32, i32})  [unwired: 1 out]
                      n3198 = property class="Tbl (严格)"(reference=w4888, "Active Cell"=w4887, "Cell BG Color"=u32 6618880) -> ()  [unwired: 1 in, 2 out]
                    }
                  }
                }
                n3199 = property on="从板号" class="DigNum (严格)"("NumText.BGColor"=u32 16777215) -> ()  [unwired: 2 in, 2 out]
                n3200 = Select(t=0, s=w4855, f=1) -> (s? t:f=w4854:i32)
                n3201 = property on="项目信息 2" class="Tbl (严格)"("Disabled"=w4854) -> ()  [unwired: 2 in, 2 out]
                n3202 = property on="加热控制参数" class="Clust (严格)"("Disabled"=2) -> ()  [unwired: 2 in, 2 out]
                n3203 = global read "功能码全局.vi" "15"() -> (w4861:bool[])
                n3204 = Index Array(array=w4861, index #1=2 ("索引"), index #2=6 ("索引")) -> (element #1=w4859:bool, element #2=w4858:bool)
                n3205 = Not(x=w4852) -> (.not. x?=w4865:bool)
              }
              frame "温度个数" {
                w4889 = FALSE ("1 6")
                n3206 = control-ref of="项目信息 2"() -> (w4900:refnum<vi>)
                n3207 = stacked-sequence {
                  tunnel: w4900 -> [w4907 w4908 w4918]
                  frame #0 {
                    n3208 = Bundle(0, 0) -> (w4906:cluster{i32, i32})  [unwired: 1 out]
                    n3209 = property class="Tbl (严格)"(reference=w4907, "Index Values"=w4906) -> ()  [unwired: 1 in, 2 out]
                  }
                  frame #1 {
                    n3210 = for {
                      N: 40 -> [_]
                      tunnel: w4908 -> [w4916]
                      i -> [w4911]
                      n3211 = Compound Arithmetic op=ADD(0 ("值"), w4911) -> (w4913:i32)
                      n3212 = Bundle(w4913, 0) -> (w4915:cluster{i32, i32})  [unwired: 1 out]
                      n3213 = property class="Tbl (严格)"(reference=w4916, "Active Cell"=w4915, "Cell BG Color"=u32 16448250) -> ()  [unwired: 1 in, 2 out]
                    }
                  }
                  frame #2 {
                    n3214 = for {
                      N: 1 -> [_]
                      tunnel: w4918 -> [w4925]
                      i -> [w4921]
                      n3215 = Add(x=1, y=w4921) -> (x+y=w4920:i32)
                      n3216 = Bundle(w4920, 0) -> (w4924:cluster{i32, i32})  [unwired: 1 out]
                      n3217 = property class="Tbl (严格)"(reference=w4925, "Active Cell"=w4924, "Cell BG Color"=u32 6618880) -> ()  [unwired: 1 in, 2 out]
                    }
                  }
                }
                n3218 = Select(t=0, s=w4892, f=1) -> (s? t:f=w4891:i32)
                n3219 = property on="项目信息 2" class="Tbl (严格)"("Disabled"=w4891) -> ()  [unwired: 2 in, 2 out]
                n3220 = property on="加热控制参数" class="Clust (严格)"("Disabled"=2) -> ()  [unwired: 2 in, 2 out]
                n3221 = property on="从板号" class="DigNum (严格)"("NumText.BGColor"=u32 16777215) -> ()  [unwired: 2 in, 2 out]
                n3222 = global read "功能码全局.vi" "15"() -> (w4898:bool[])
                n3223 = Index Array(array=w4898, index #1=3 ("索引"), index #2=7 ("索引")) -> (element #1=w4896:bool, element #2=w4895:bool)
                n3224 = Not(x=w4889) -> (.not. x?=w4902:bool)
              }
              frame "SOC过低", "电压不均衡", "电压过低", "电压过高", "温度不均衡", "温度过低", "温度过高", "一级故障阀值" {
                w4926 = FALSE ("1 6")
                n3225 = property on="从板号" class="DigNum (严格)"("NumText.BGColor"=u32 16777215) -> ()  [unwired: 2 in, 2 out]
                n3226 = Select(t=0, s=w4928, f=1) -> (s? t:f=w4929:i32)
                n3227 = property on="一级故障 6" class="Clust (严格)"("DisabledEnum"=w4929) -> ()  [unwired: 2 in, 2 out]
                n3228 = global read "功能码全局.vi" "18"() -> (w4935:bool[])
                n3229 = Index Array(array=w4935, index #1=2 ("索引"), index #2=5 ("索引")) -> (element #1=w4933:bool, element #2=w4932:bool)
                n3230 = Not(x=w4926) -> (.not. x?=w4937:bool)
              }
              frame "SOC过低(2)", "电压不均衡(2)", "电压过低(2)", "电压过高(2)", "二级故障阀值", "温度不均衡(2)", "温度过低(2)", "温度过高(2)" {
                w4939 = FALSE ("1 6")
                n3231 = property on="从板号" class="DigNum (严格)"("NumText.BGColor"=u32 16777215) -> ()  [unwired: 2 in, 2 out]
                n3232 = Select(t=0, s=w4942, f=1) -> (s? t:f=w4941:i32)
                n3233 = property on="一级故障 7" class="Clust (严格)"("DisabledEnum"=w4941) -> ()  [unwired: 2 in, 2 out]
                n3234 = global read "功能码全局.vi" "18"() -> (w4948:bool[])
                n3235 = Index Array(array=w4948, index #1=3 ("索引"), index #2=6 ("索引")) -> (element #1=w4946:bool, element #2=w4945:bool)
                n3236 = Not(x=w4939) -> (.not. x?=w4950:bool)
              }
              frame "SOC过低(3)", "电压不均衡(3)", "电压过低(3)", "电压过高(3)", "三级故障阀值", "温度不均衡(3)", "温度过低(3)", "温度过高(3)" {
                w4952 = FALSE ("1 6")
                n3237 = property on="从板号" class="DigNum (严格)"("NumText.BGColor"=u32 16777215) -> ()  [unwired: 2 in, 2 out]
                n3238 = Select(t=0, s=w4955, f=1) -> (s? t:f=w4954:i32)
                n3239 = property on="一级故障 8" class="Clust (严格)"("DisabledEnum"=w4954) -> ()  [unwired: 2 in, 2 out]
                n3240 = global read "功能码全局.vi" "18"() -> (w4961:bool[])
                n3241 = Index Array(array=w4961, index #1=4 ("索引"), index #2=7 ("索引")) -> (element #1=w4959:bool, element #2=w4958:bool)
                n3242 = Not(x=w4952) -> (.not. x?=w4963:bool)
              }
              frame "快换参数" {
                w4965 = FALSE ("1 6")
                n3243 = Select(t=0, s=w4986, f=1) -> (s? t:f=w4985:i32)
                n3244 = property on="电池组信息" class="Clust (严格)"("Disabled"=w4985) -> ()  [unwired: 2 in, 2 out]
                n3245 = property on="从板号" class="DigNum (严格)"("NumText.BGColor"=u32 16777215) -> ()  [unwired: 2 in, 2 out]
                n3246 = global read "功能码全局.vi" "24"() -> (w4982:bool[])
                n3247 = global read "功能码全局.vi" "23"() -> (w4983:bool[])
                n3248 = Index Array(array=w4982) -> (element #3=w4972:bool, element #4=w4971:bool, element #5=w4970:bool, element #6=w4969:bool, element #7=w4968:bool, element #8=w4967:bool)  [unwired: 8 in, 2 out]
                n3249 = Index Array(array=w4983) -> (element #3=w4981:bool, element #4=w4980:bool, element #5=w4979:bool, element #6=w4978:bool, element #7=w4977:bool, element #8=w4976:bool)  [unwired: 8 in, 2 out]
                n3250 = Build Array(w4972, w4971, w4970, w4969, w4968, w4967) -> (w4973:bool[])
                n3251 = Build Array(w4981, w4980, w4979, w4978, w4977, w4976) -> (w4975:bool[])
                n3252 = And Array Elements(Boolean array=w4973) -> (logical AND=w4966:bool)
                n3253 = And Array Elements(Boolean array=w4975) -> (logical AND=w4974:bool)
                n3254 = Not(x=w4965) -> (.not. x?=w4989:bool)
              }
              frame "电池包信息1" {
                w4994 = 2
                w5002 = 2
                w4993 = 2
                w4991 = FALSE ("1 6")
                n3255 = Select(t=0, s=w4999, f=1) -> (s? t:f=w4992:i32)
                n3256 = property on="串联数" class="DigNum (严格)"("Disabled"=w4992) -> ()  [unwired: 2 in, 2 out]
                n3257 = property on="并联数" class="DigNum (严格)"("Disabled"=w4992) -> ()  [unwired: 2 in, 2 out]
                n3258 = property on="电池厂家" class="DigNum (严格)"("Disabled"=w4992) -> ()  [unwired: 2 in, 2 out]
                n3259 = property on="电池类型" class="DigNum (严格)"("Disabled"=w4992) -> ()  [unwired: 2 in, 2 out]
                n3260 = property on="额定能量" class="DigNum (严格)"("Disabled"=w4992) -> ()  [unwired: 2 in, 2 out]
                n3261 = property on="额定容量" class="DigNum (严格)"("Disabled"=w4992) -> ()  [unwired: 2 in, 2 out]
                n3262 = property on="实际容量" class="DigNum (严格)"("Disabled"=w4992) -> ()  [unwired: 2 in, 2 out]
                n3263 = property on="电池组信息" class="Clust (严格)"("Disabled"=w4992) -> ()  [unwired: 2 in, 2 out]
                n3264 = property on="生产日期" class="Str"("DisabledEnum"=w4992) -> ()  [unwired: 2 in, 2 out]
                n3265 = property on="车牌号" class="Str"("DisabledEnum"=w4993) -> ()  [unwired: 2 in, 2 out]
                n3266 = property on="产权标识" class="DigNum (严格)"("Disabled"=w4992) -> ()  [unwired: 2 in, 2 out]
                n3267 = property on="应用车型" class="DigNum (严格)"("Disabled"=w4992) -> ()  [unwired: 2 in, 2 out]
                n3268 = property on="额定总压" class="DigNum (严格)"("Disabled"=w4992) -> ()  [unwired: 2 in, 2 out]
                n3269 = property on="电池包序号" class="DigNum (严格)"("DisabledEnum"=w4992) -> ()  [unwired: 2 in, 2 out]
                n3270 = property on="电池包组号" class="DigNum (严格)"("DisabledEnum"=w4993) -> ()  [unwired: 2 in, 2 out]
                n3271 = property on="最大允许单体电压" class="DigNum (严格)"("Disabled"=w5002) -> ()  [unwired: 2 in, 2 out]
                n3272 = property on="最大允许总电压" class="DigNum (严格)"("Disabled"=w5002) -> ()  [unwired: 2 in, 2 out]
